vi "ROI group-Create new ROI Group.vi"(11 "Save?":bool=TRUE) -> (0 "error out":errorcluster, 1 "New group setup":T1 {"Group region specifier cluster"."Contours"."Type" items=["No Selection", "Point", "Line", "Rectangle", "Oval", "Polygon", "Freehand Region", "Annulus", "Unused2", "Unused3", "Broken Line", "Freehand Line", "Rotated Rectangle"]})   [LabVIEW 2020]
uses:
  ROI Selection Interface/ROI group info cluster.ctl
  Experiment header interface/Typedefs/Save-Load-Save as-Load last enum.ctl
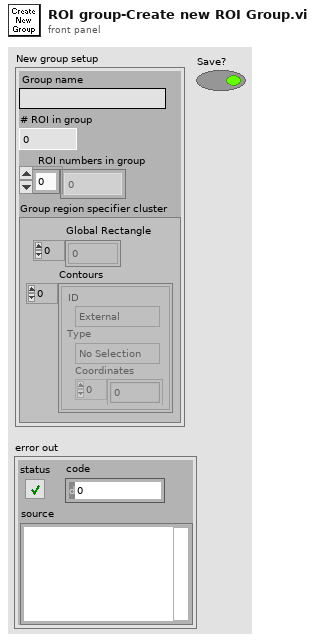
[diagram p1: front panel]
types:
  T1 = typedef "ROI group info cluster.ctl" = cluster{"Group name":string, "# ROI in group":i32, "ROI numbers in group":i32[], "Group region specifier cluster":T2}
  T2 = typedef "ROI Descriptor" = cluster{"Global Rectangle":i32[], "Contours":cluster{"ID":enum32{"External", "Internal"}, "Type":u32, "Coordinates":i32[]}[]}
  T3 = enum8{"Enabled", "Disabled", "Disabled and Grayed Out"}
  T4 = typedef "Save-Load-Save as-Load last enum.ctl" = enum16{"Save file", "Save file as", "Load file", "Load last file"}
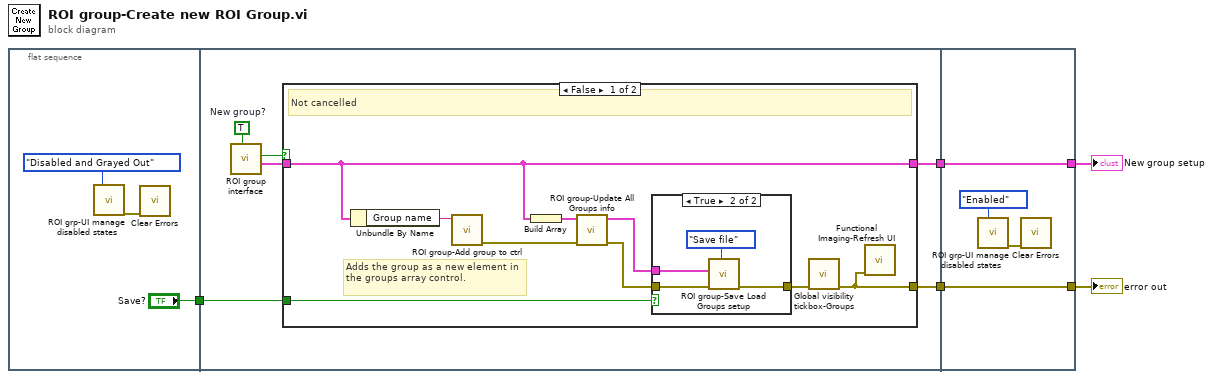
[diagram p0: block diagram]
diagram:
  n1 = flat-sequence {
    tunnel: ["Save?"] -> w1
    tunnel: [w13] -> w3
    tunnel: [w11] -> w2
    tunnel: w1 -> [w9]
    tunnel: [w31] -> w4
    tunnel: [w32] -> w5
    tunnel: w3 -> [w32]
    tunnel: w2 -> [w31]
    frame #0 {
      n2 = call "ROI grp-UI manage disabled states.vi"("UI elemente enabled?"=T3."Disabled and Grayed Out") -> ("error out"=w8:errorcluster)  [unwired: 10 in]
      n3 = call <vilib>:"Clear Errors.vi"("error in (no error)"=w8) -> ()  [unwired: 5 in, 2 out]
    }
    frame #1 {
      w10 = TRUE  # New group?
      n4 = call "ROI group interface.vi"("New group (F)"=w10) -> ("POI group info cluster"=w14:T1, "Cancelled"=w12:bool)  [unwired: 8 in, 1 out]
      n5 = case shown="False" w12 {
        tunnel: w14 -> [w21 _]
        tunnel: [w15 _] -> w11
        tunnel: [w21 _] -> w13
        tunnel: w9 -> [w17 _]
        frame False {
          # "Adds the group as a new element in the groups array control."
          # "Not cancelled"
          n6 = Unbundle By Name(w21) -> ("Group name"=w18:string)
          n7 = call "ROI group-Add group to ctrl.vi"("Group Name"=w18) -> ("error out"=w20:errorcluster)  [unwired: 10 in]
          n8 = Build Array(w21) -> (w22:T1[])
          n9 = call "ROI group-Update All Groups info.vi"("error in (no error)"=w20, "Groups setup to add/update"=w22) -> ("error out"=w19:errorcluster, "Updated \"All groups\" setup"=w23:T1[])  [unwired: 8 in]
          n10 = case shown="True" w17 {
            tunnel: w23 -> [_ w27]
            tunnel: w19 -> [w24 w26]
            tunnel: [w24 w25] -> w16
            frame False {
            }
            frame True {
              n11 = call "ROI group-Save Load Groups setup.vi"("error in (no error)"=w26, "Function"=Save-Load-Save_as-Load_last_enum."Save file", "Groups setup to save"=w27) -> ("error out"=w25:errorcluster)  [unwired: 7 in, 1 out]
            }
          }
          n12 = call "Global visibility tickbox-Groups.vi"("error in (no error)"=w16) -> ("error out"=w15:errorcluster)  [unwired: 10 in]
          n13 = call "Functional Imaging-Refresh UI.vi"("error in (no error)"=w15) -> ()  [unwired: 11 in]
        }
        frame True {
          # "Cancelled"
        }
      }
    }
    frame #2 {
      n14 = call "ROI grp-UI manage disabled states.vi"("UI elemente enabled?"=T3."Enabled") -> ("error out"=w29:errorcluster)  [unwired: 10 in]
      n15 = call <vilib>:"Clear Errors.vi"("error in (no error)"=w29) -> ()  [unwired: 5 in, 2 out]
    }
  }
  "error out" <- w4
  "New group setup" <- w5
